vi "Render.vi"(8 "error in (no error)":errorcluster, 11 "XRay CArm in":refnum<class "XRay CArm.lvclass">=refnum) -> (0 "error out":errorcluster, 2 "Scene Object":refnum<vi>, 3 "XRay CArm out":refnum<class "XRay CArm.lvclass">)   [LabVIEW 2026, in "XRay CArm.lvclass"]
uses:
  XRay CArm.lvclass
  XRay CArm.lvclass/XRay CArm.ctl
  <vilib>/picture/3D Picture Control/Object/Add Object (reference).vi
  <vilib>/picture/3D Picture Control/NI_3D Picture Control.lvlib
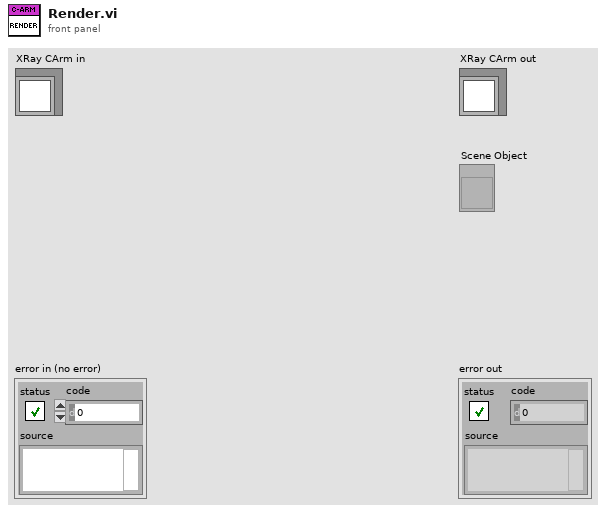
[diagram p1: front panel]
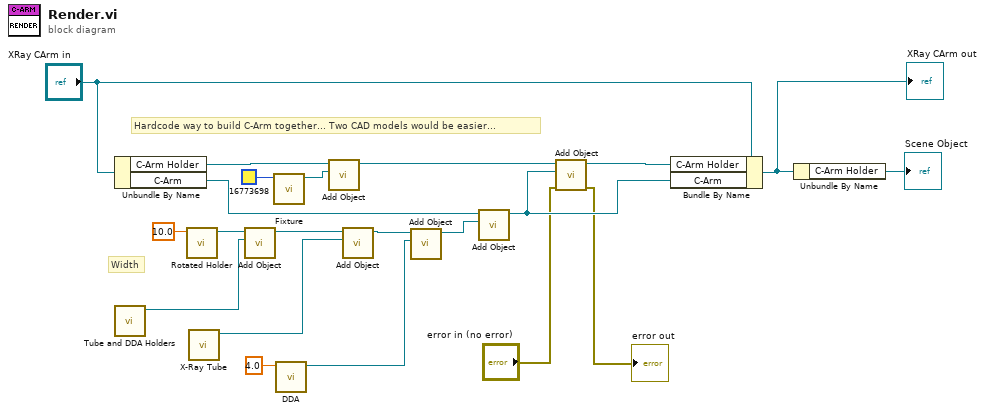
[diagram p0: block diagram]
diagram:
  # "Hardcode way to build C-Arm together... Two CAD models would be easier..."
  # "Width"
  n1 = Unbundle By Name("XRay CArm in") -> ("C-Arm Holder"=w9:refnum<vi>, "C-Arm"=w18:refnum<vi>)
  n2 = call "Tube and DDA Holders.vi"() -> ("SceneObject out"=w5:refnum<vi>)  [unwired: 10 in, 1 out]
  n3 = call "Rotated Holder.vi"("Box Length Y 3"=sgl 10.0) -> ("SceneObject out"=w10:refnum<vi>)  [unwired: 9 in, 1 out]
  n4 = call "X-Ray Tube.vi"() -> ("SceneObject out"=w11:refnum<vi>)  [unwired: 10 in, 1 out]
  n5 = call-poly <vilib>:"Add Object.vi"("New Object In"=w5, "Scene Object In"=w10) -> ("Scene Object Out"=w6:refnum<vi>)  [unwired: 7 in, 2 out]
  n6 = call "Fixture.vi"("Color"=u32 16773698) -> ("SceneObject out"=w8:refnum<vi>)  [unwired: 9 in, 1 out]
  n7 = call "DDA.vi"("Box Length X (4)"=sgl 4.0 ("Box Length X")) -> ("SceneObject out"=w13:refnum<vi>)  [unwired: 9 in, 1 out]
  n8 = call-poly <vilib>:"Add Object.vi"("New Object In"=w8, "Scene Object In"=w9) -> ("Scene Object Out"=w17:refnum<vi>)  [unwired: 7 in, 2 out]
  n9 = call-poly <vilib>:"Add Object.vi"("New Object In"=w11, "Scene Object In"=w6) -> ("Scene Object Out"=w14:refnum<vi>)  [unwired: 7 in, 2 out]
  n10 = call-poly <vilib>:"Add Object.vi"("New Object In"=w13, "Scene Object In"=w14) -> ("Scene Object Out"=w12:refnum<vi>)  [unwired: 7 in, 2 out]
  n11 = call-poly <vilib>:"Add Object.vi"("New Object In"=w12, "Scene Object In"=w18) -> ("Scene Object Out"=w16:refnum<vi>)  [unwired: 7 in, 2 out]
  n12 = call-poly <vilib>:"Add Object.vi"("error in (no error)"="error in (no error)", "New Object In"=w16, "Scene Object In"=w17) -> ("error out"=→"error out":errorcluster, "Scene Object Out"=w15:refnum<vi>)  [unwired: 6 in, 1 out]
  n13 = Bundle By Name(cluster="XRay CArm in", "C-Arm Holder"=w15, "C-Arm"=w16) -> (w4:refnum<class "XRay CArm.lvclass">)
  "XRay CArm out" <- w4
  n14 = Unbundle By Name(w4) -> ("C-Arm Holder"=→"Scene Object":refnum<vi>)
